vi "setAmplitude.vi"(8 "error in (no error)":errorcluster, 10 "Voltage Pk-Pk":dbl, 11 "VISA resource name":refnum<visa-resource-name>) -> (0 "error out":errorcluster, 3 "VISA resource name out":refnum<visa-resource-name>)   [LabVIEW 2023, in "Keysight-33500B.lvlib"]
doc: "<b>Author:</b> Wolfgang\n<b>Description:</b> >>>> Set Amplitude Vpk>>>"
uses:
  Keysight-33500B.lvlib
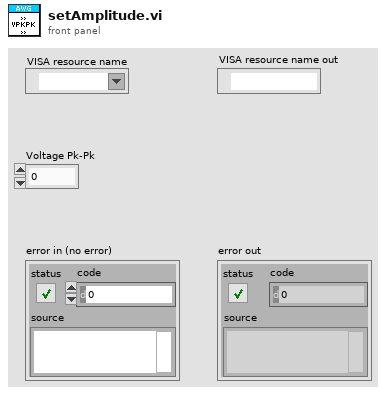
[diagram p1: front panel]
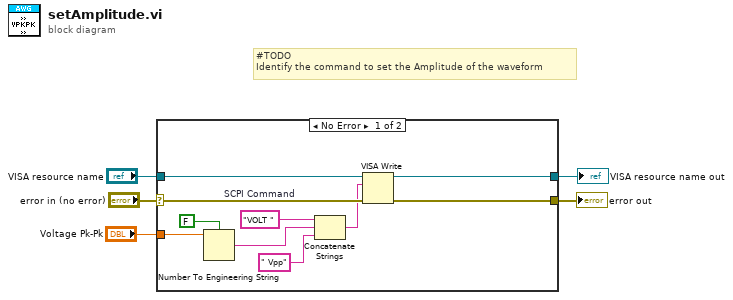
[diagram p0: block diagram]
diagram:
  # "#TODO\nIdentify the command to set the Amplitude of the waveform"
  n1 = case shown="No Error" "error in (no error)" {
    selector: "error in (no error)" -> [w14 w17]
    tunnel: [w9 w16] -> w5
    tunnel: [w8 w17] -> w3
    tunnel: "VISA resource name" -> [w15 w16]
    tunnel: "Voltage Pk-Pk" -> [w13 _]
    frame No Error {
      w11 = "VOLT "  # SCPI Command
      n2 = Number To Engineering String(1:FALSE ("use system decimal point (T)"), 4:w13) -> (0:w10:string)  [unwired: 2 in]
      n3 = Concatenate Strings(w11, w10, " Vpp" ("string")) -> (w12:string)
      n4 = VISA Write(VISA resource name=w15, write buffer=w12, error in (no error)=w14) -> (VISA resource name out=w9:refnum<visa-resource-name>, error out=w8:errorcluster)  [unwired: 1 out]
    }
    frame Error {
    }
  }
  "VISA resource name out" <- w5
  "error out" <- w3
